vi "Retrieve Sample from Container.vi"(7 "Message Priority (Normal)":T1=enum."Normal", 8 "error in (no error)":errorcluster, 9 "timeout in ms (1000)":i32=1000, 10 "Sample Container":T2, 11 "cRIO-CO2 in":refnum<class "cRIO-CO2.lvclass">) -> (0 "error out":errorcluster, 1 "timed out?":bool, 2 "Sample.lvclass":refnum<class "Sample.lvclass">, 3 "cRIO-CO2 out":refnum<class "cRIO-CO2.lvclass">, 4 "Valid Sample (Not Empry nor Dirt)":bool)   [LabVIEW 2015, in "cRIO-Carbondioxide.lvlib" / "cRIO-CO2.lvlib" / "cRIO-CO2.lvclass"]
uses:
  cRIO-CO2.lvclass
  Controls/Sample Transfer Container Enumerator.ctl
  subs/Sample/Sample.lvclass
  <vilib>/ActorFramework/Message Enqueuer/Message Priority.ctl
  CO2 Actor Messages/Read Sample from Container Msg/Read Sample from Container Msg.lvclass
  CO2 Actor Messages/Read Sample from Container Msg/Read Sample from Container Msg.lvclass/Read Sample from Container Msg.ctl
  cRIO-CO2.lvclass/cRIO-CO2.ctl
  <vilib>/ActorFramework/Reply Msg/Reply Msg.lvclass/Reply Msg.ctl
  <vilib>/ActorFramework/Message Enqueuer/Message Enqueuer.lvclass/Message Enqueuer.ctl
  subs/Sample/Sample.lvclass/Sample.ctl
  <vilib>/ActorFramework/Message Enqueuer/Enqueue.vi
  <vilib>/ActorFramework/Message Priority Queue/Priority Enqueue.vi
  <vilib>/ActorFramework/Reply Msg/Reply Msg.lvclass
  <vilib>/ActorFramework/Message Enqueuer/Message Enqueuer.lvclass
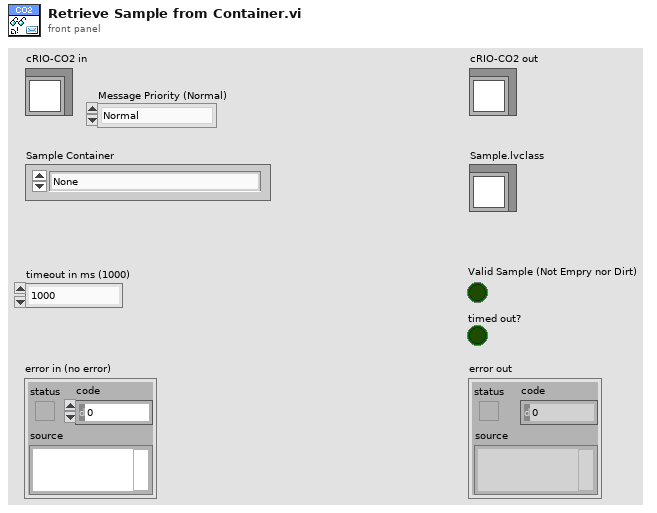
[diagram p1: front panel]
types:
  T1 = typedef "Actor Framework.lvlib/Message Enqueuer.lvclass/Message Priority.ctl" = enum16{"Low", "Normal", "High"}
  T2 = typedef "Sample Transfer Container Enumerator.ctl" = enum16{"None", "Sample 1", "Sample 2", "Sample 3", "Sample 4", "Sample 5", "Storage 01", "Storage 02", "Storage 03", "Storage 04", "Storage 05", "Storage 06", "Storage 07", "Storage 08", "Storage 09", "Storage 10", "Storage 11", "Storage 12", "Syringe", "Undefined"}
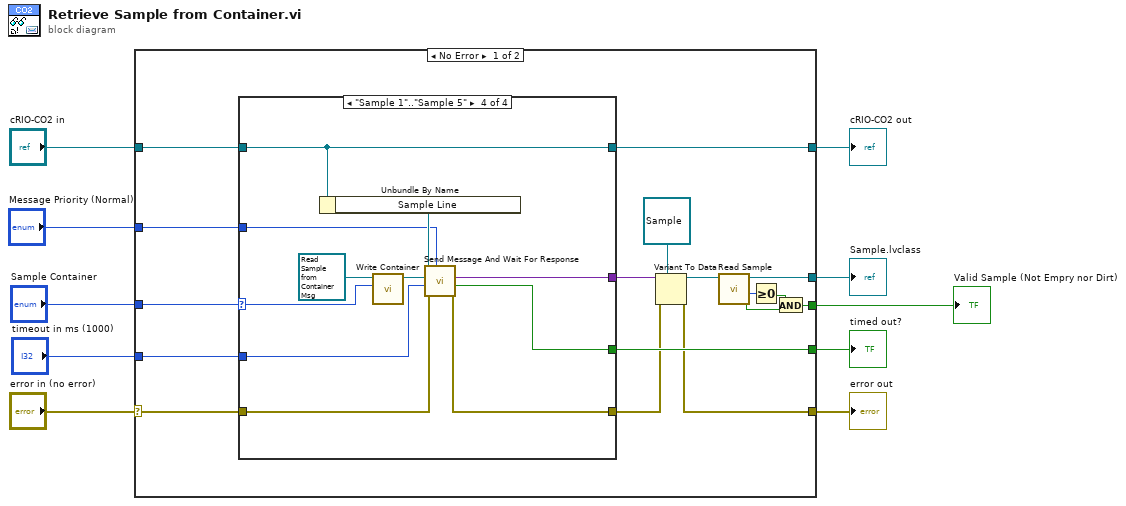
[diagram p0: block diagram]
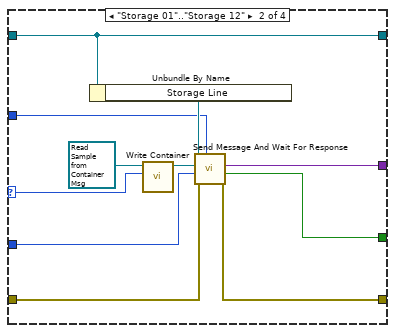
[diagram p3: hidden frame]
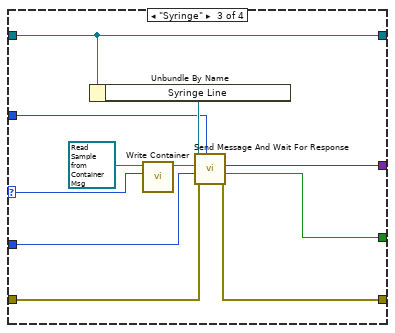
[diagram p4: hidden frame]
diagram:
  n1 = case shown="No Error" "error in (no error)" {
    selector: "error in (no error)" -> [w26 w64]
    tunnel: [w17 w64] -> w9
    tunnel: [w23 w63] -> w7
    tunnel: "cRIO-CO2 in" -> [w24 w63]
    tunnel: "Sample Container" -> [w27 _]
    tunnel: "timeout in ms (1000)" -> [w25 _]
    tunnel: [w22 _] -> w4
    tunnel: "Message Priority (Normal)" -> [w21 _]
    tunnel: [w15 _] -> w2
    tunnel: [w11 _] -> w1
    frame No Error {
      n2 = case shown="\"Sample 1\"..\"Sample 5\"" w27 {
        selector: w27 -> [_ w38 w49 w60]
        tunnel: w26 -> [w28 w37 w48 w59]
        tunnel: w25 -> [_ w36 w47 w58]
        tunnel: w24 -> [w29 w35 w46 w57]
        tunnel: [w29 w35 w46 w57] -> w23
        tunnel: [w28 w33 w44 w55] -> w18
        tunnel: [_ w32 w43 w54] -> w20
        tunnel: [_ w31 w42 w53] -> w22
        tunnel: w21 -> [_ w30 w41 w52]
        frame "None", "Undefined" {
        }
        frame "Storage 01".."Storage 12" {
          n3 = Unbundle By Name(w35) -> ("Storage Line"=w34:refnum<class "Message Enqueuer.lvclass">)
          n4 = call "Write Container.vi"("Sample Transfer Container"=w38, "Read Sample from Container Msg in"=refnum<class "Read Sample from Container Msg.lvclass"> refnum ("cRIO-Carbondioxide.lvlib:CO2-Actor.lvlib:Read Sample from Container Msg.lvclass")) -> ("Read Sample from Container Msg out"=w39:refnum<class "Read Sample from Container Msg.lvclass">)  [unwired: 9 in]
          n5 = call <vilib>:"Send Message And Wait For Response.vi"("Message Priority (Normal)"=w30, "error in (no error)"=w37, "timeout in ms (-1)"=w36, "Original Message"=w39, "Message Enqueuer in"=w34) -> ("error out"=w33:errorcluster, "timed out?"=w31:bool, "Reply"=w32:variant)  [unwired: 3 in, 1 out]
        }
        frame "Syringe" {
          n6 = Unbundle By Name(w46) -> ("Syringe Line"=w45:refnum<class "Message Enqueuer.lvclass">)
          n7 = call "Write Container.vi"("Sample Transfer Container"=w49, "Read Sample from Container Msg in"=refnum<class "Read Sample from Container Msg.lvclass"> refnum ("cRIO-Carbondioxide.lvlib:CO2-Actor.lvlib:Read Sample from Container Msg.lvclass")) -> ("Read Sample from Container Msg out"=w50:refnum<class "Read Sample from Container Msg.lvclass">)  [unwired: 9 in]
          n8 = call <vilib>:"Send Message And Wait For Response.vi"("Message Priority (Normal)"=w41, "error in (no error)"=w48, "timeout in ms (-1)"=w47, "Original Message"=w50, "Message Enqueuer in"=w45) -> ("error out"=w44:errorcluster, "timed out?"=w42:bool, "Reply"=w43:variant)  [unwired: 3 in, 1 out]
        }
        frame "Sample 1".."Sample 5" {
          n9 = Unbundle By Name(w57) -> ("Sample Line"=w56:refnum<class "Message Enqueuer.lvclass">)
          n10 = call "Write Container.vi"("Sample Transfer Container"=w60, "Read Sample from Container Msg in"=refnum<class "Read Sample from Container Msg.lvclass"> refnum ("cRIO-Carbondioxide.lvlib:CO2-Actor.lvlib:Read Sample from Container Msg.lvclass")) -> ("Read Sample from Container Msg out"=w61:refnum<class "Read Sample from Container Msg.lvclass">)  [unwired: 9 in]
          n11 = call <vilib>:"Send Message And Wait For Response.vi"("Message Priority (Normal)"=w52, "error in (no error)"=w59, "timeout in ms (-1)"=w58, "Original Message"=w61, "Message Enqueuer in"=w56) -> ("error out"=w55:errorcluster, "timed out?"=w53:bool, "Reply"=w54:variant)  [unwired: 3 in, 1 out]
        }
      }
      n12 = Variant To Data(error in=w18, type=refnum<class "Sample.lvclass"> refnum ("Sample.lvclass"), Variant=w20) -> (data=w16:refnum<class "Sample.lvclass">, error out=w17:errorcluster)
      n13 = call "Read Sample.vi"("Sample in"=w16) -> ("Sample In"=w12:bool, "Ti Cathode"=w14:i8, "Sample out"=w15:refnum<class "Sample.lvclass">)  [unwired: 6 in, 2 out]
      n14 = Greater Or Equal To 0?(x=w14) -> (x >= 0?=w13:bool)
      n15 = And(x=w13, y=w12) -> (x .and. y?=w11:bool)
    }
    frame Error {
    }
  }
  "error out" <- w9
  "cRIO-CO2 out" <- w7
  "Sample.lvclass" <- w2
  "Valid Sample (Not Empry nor Dirt)" <- w1
  "timed out?" <- w4
